vi "_interfacebrowser build tree table in CSM mode.vi"(6 "Config Path":path, 8 "Error in":errorcluster caption="Error in (no error)") -> (0 "Error out":errorcluster, 2 "Type":string[](array[string]), 3 "Tree Table":string[][](array[string]))   [LabVIEW 2017]
uses:
  _csmHelper/API with lvcsm Support/CSM-Helper API with lvcsm Support.lvlib
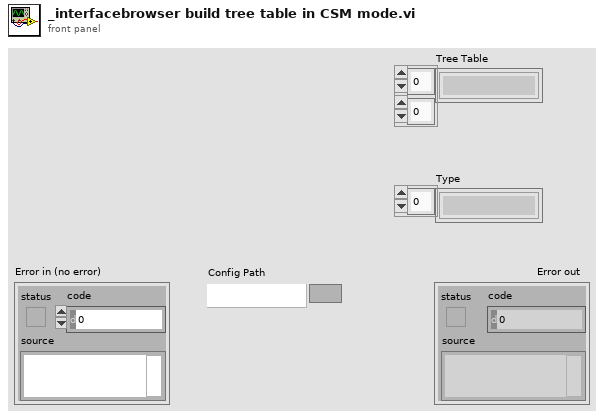
[diagram p1: front panel]
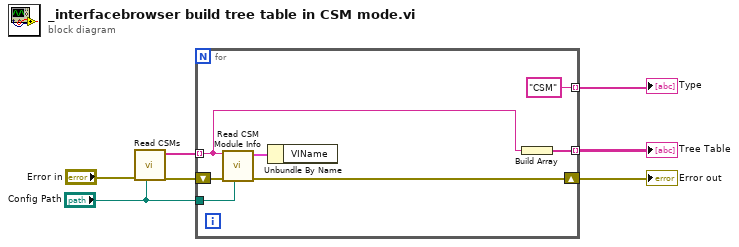
[diagram p0: block diagram]
diagram:
  n1 = call "Read CSMs.vi"("Config Path"="Config Path", "Error in"="Error in") -> ("Error out"=w5:errorcluster, "Array"=w4:string[])  [unwired: 8 in]
  n2 = for {
    tunnel: w4 -> [w13] mode=indexing
    tunnel: [w12] -> w6 mode=indexing
    tunnel: ["CSM" ("Delimiter")] -> w7 mode=indexing
    shift-right: [w8] -> w2
    shift-left: w5 -> [w11]
    tunnel: "Config Path" -> [w9]
    n3 = call "Read CSM Module Info.vi"("Config Path"=w9, "error in (no error)"=w11, "CSM Name"=w13) -> ("error out"=w8:errorcluster, "Cluster"=w14:cluster{"VIName":string})  [unwired: 7 in]
    n4 = Unbundle By Name(w14) -> ()  [unwired: 1 out]
    n5 = Build Array(w13) -> (w12:string[])
  }
  "Type" <- w7
  "Tree Table" <- w6
  "Error out" <- w2
